vi "replaceTypeToken.vi"(8 "error in (no error)":errorcluster, 10 "Query In":string, 11 "Banking Transaction in":refnum<class "Banking Transaction.lvclass">) -> (0 "error out":errorcluster, 2 "Query Out":string, 3 "Banking Transaction out":refnum<class "Banking Transaction.lvclass">)   [LabVIEW 2018, in "Banking Transaction.lvclass"]
uses:
  Banking Transaction.lvclass
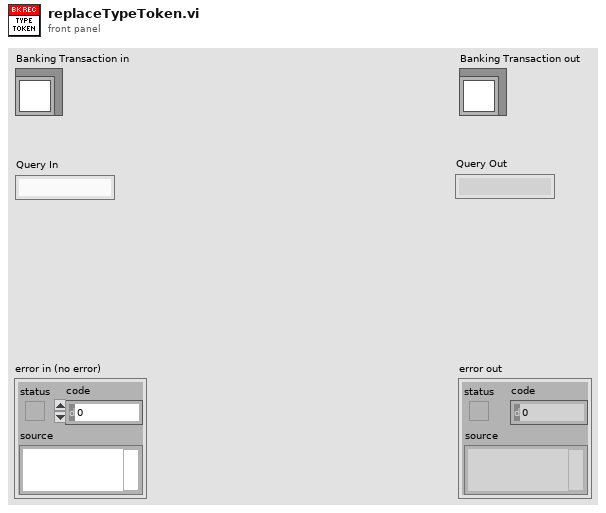
[diagram p1: front panel]
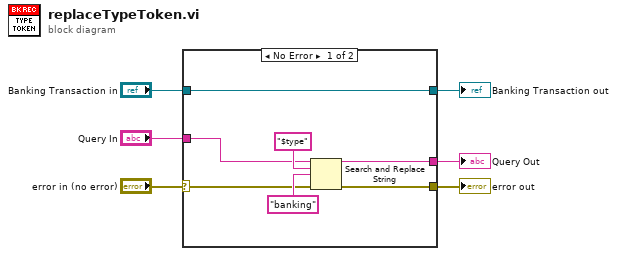
[diagram p0: block diagram]
diagram:
  n1 = case shown="No Error" "error in (no error)" {
    selector: "error in (no error)" -> [w7 w14]
    tunnel: [w9 w15] -> w6
    tunnel: "Query In" -> [w8 _]
    tunnel: "Banking Transaction in" -> [w9 w15]
    tunnel: [w13 w14] -> w3
    tunnel: [w12 _] -> w2
    frame No Error {
      n2 = Search and Replace String(input string=w8, search string="$type", replace string="banking" ("replace string (\"\")"), error in=w7) -> (result string=w12:string, error out=w13:errorcluster)  [unwired: 4 in, 2 out]
    }
    frame Error {
    }
  }
  "error out" <- w3
  "Banking Transaction out" <- w6
  "Query Out" <- w2
